vi "Channel spliter.vi"(11 "image data":T1) -> (1 "Array 2":u8[][](array[numeric]), 2 "Array":u8[][](array[numeric]), 3 "Array 3":u8[][](array[numeric]), 4 "right":i16, 5 "bottom":i16)   [LabVIEW 2016]
uses:
  <vilib>/picture/picture.llb/imagedata.ctl
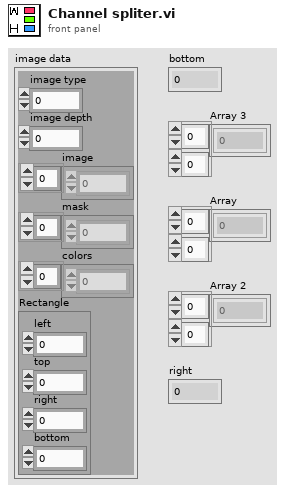
[diagram p1: front panel]
types:
  T1 = typedef "imagedata.ctl" = cluster{"image type":i32, "image depth":i32, "image":u8[], "mask":u8[], "colors":u32[], "Rectangle":cluster{"left":i16, "top":i16, "right":i16, "bottom":i16}}
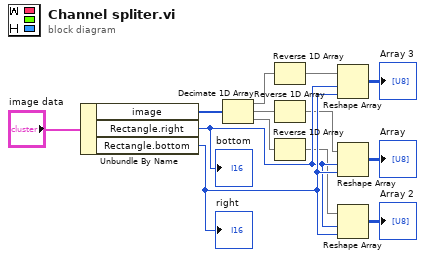
[diagram p0: block diagram]
diagram:
  n1 = Unbundle By Name("image data") -> ("image"=w8:u8[], "Rectangle.right"=w7:i16, "Rectangle.bottom"=w13:i16)
  "right" <- w13
  "bottom" <- w7
  n2 = Decimate 1D Array(w8) -> (w6:u8[], w4:u8[], w2:u8[])
  n3 = Reverse 1D Array(array=w6) -> (reversed array=w5:u8[])
  n4 = Reverse 1D Array(array=w4) -> (reversed array=w3:u8[])
  n5 = Reverse 1D Array(array=w2) -> (reversed array=w1:u8[])
  n6 = Reshape Array(w5, w7, w13) -> (→"Array 3":u8[][])
  n7 = Reshape Array(w3, w7, w13) -> (→"Array":u8[][])
  n8 = Reshape Array(w1, w7, w13) -> (→"Array 2":u8[][])
